vi "Init Logger.vi"(8 "error in (no error)":errorcluster, 10 "File Send Interval (Seconds)":dbl=600.0) -> (0 "error out":errorcluster, 3 "Logger out.lvclass":refnum<class "Logger.lvclass">)   [LabVIEW 2019, in "Logger.lvclass"]
uses:
  Logger.lvclass
  <vilib>/Skyline/Tag/Wrapper/Wrapper_class/Tag Value Cluster Wrapper.ctl
  <vilib>/Skyline/Configuration/Configuration_class/NI Skyline Configuration.lvclass
  <vilib>/Skyline/Tag/Shared/typedefs/Tag Value Cluster.ctl
  <vilib>/Skyline/Tag/Shared/typedefs/DataType.ctl
  <vilib>/Skyline/Tag/Wrapper/Wrapper_class/NI Skyline Tag.lvclass
  <vilib>/Skyline/Tag/Shared/typedefs/TagProperty.ctl
  Logger.lvclass/Logger.ctl
  <vilib>/Skyline/Tag/Wrapper/Wrapper AMQP_class/Open Tag AMQP.vi
  <vilib>/Skyline/Tag/Wrapper/Wrapper_class/Generate Tag Cluster (String) 2.vi
  <vilib>/Skyline/Tag/Wrapper/Wrapper_class/Generate Tag Cluster (Boolean) 2.vi
  <vilib>/Skyline/Tag/Wrapper/Wrapper_class/Generate Tag Cluster (I32) 2.vi
  <vilib>/Skyline/Message/AMQP/sync/Open (Sync).vi
  <vilib>/Skyline/Message/AMQP/NI Skyline Message AMQP (Sync).lvclass
  <vilib>/Skyline/Tag/Shared/NI Skyline Tag.lvlib
  <vilib>/Skyline/Tag/Wrapper/Wrapper AMQP_class/NI Skyline Tag AMQP.lvclass
  <vilib>/Skyline/Message/NI Skyline Message.lvclass
  <vilib>/Skyline/Utilities/NI Skyline Utilities.lvlib
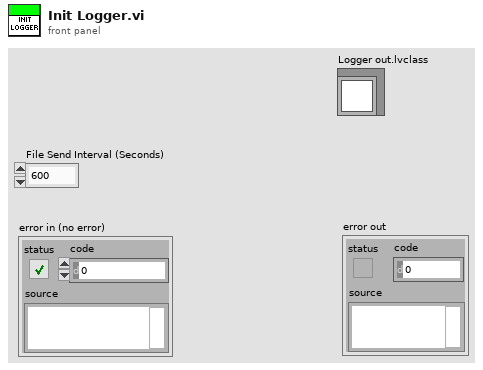
[diagram p1: front panel]
types:
  T1 = typedef "NI Skyline Tag.lvclass/Tag Value Cluster Wrapper.ctl" = cluster{"Configuration":refnum<class "NI Skyline Configuration.lvclass">, "Tag Cluster":T2}
  T2 = typedef "NI Skyline Tag.lvlib/Tag Value Cluster.ctl" = cluster{"Path":string, "Data Type":T3, "Value":string, "Time Stamp":timestamp}
  T3 = typedef "NI Skyline Tag.lvlib/DataType.ctl" = enum32{"Double", "I32", "String", "Boolean", "U64", "Timestamp"}
  T4 = typedef "NI Skyline Tag.lvlib/TagProperty.ctl" = cluster{"key":string, "value":string}
  T5 = cluster{"Tag Units":string, "Tag Path":string, "Tag Reference":refnum<class "NI Skyline Tag.lvclass">}
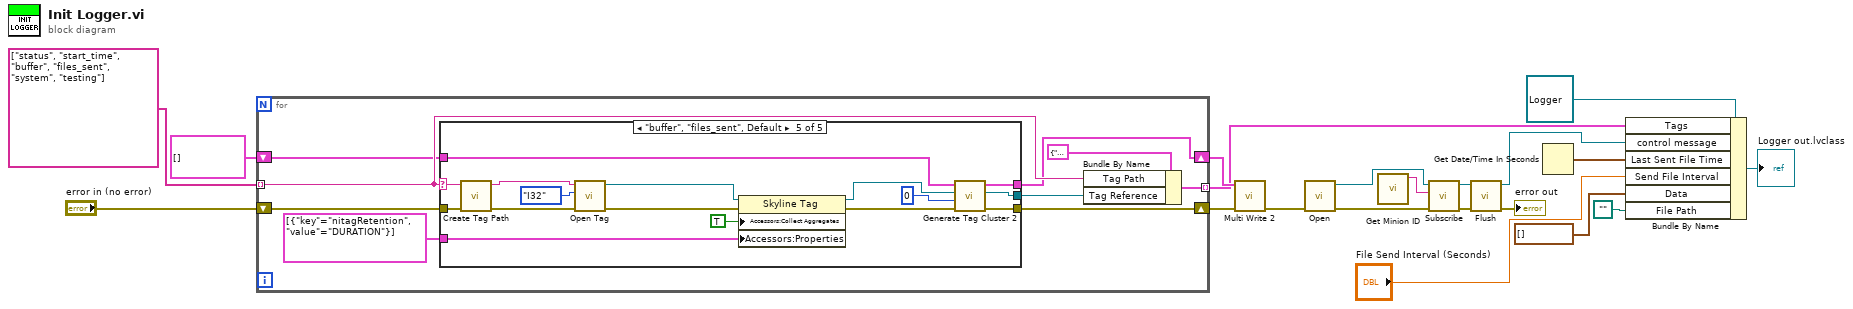
[diagram p0: block diagram]
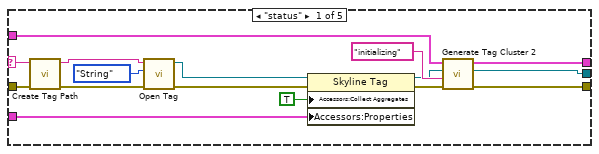
[diagram p2: hidden frame]
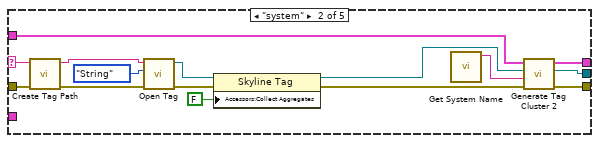
[diagram p3: hidden frame]
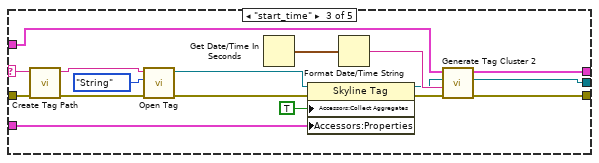
[diagram p4: hidden frame]
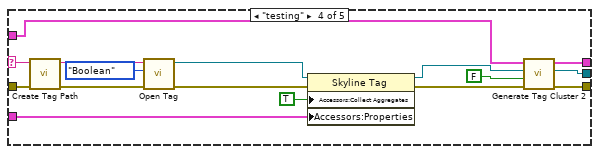
[diagram p5: hidden frame]
diagram:
  n1 = for {
    shift-right: [w29] -> w15
    shift-left: "error in (no error)" -> [w26]
    tunnel: string[] ["status", "start_time", "buffer", "files_sent", "system", "testing"] -> [w27] mode=indexing
    tunnel: [w28] -> w3 mode=indexing
    shift-right: [w22] -> w10
    shift-left: T1[] [] ("tag clusters out") -> [w23]
    n2 = case shown="\"buffer\", \"files_sent\", Default" w27 {
      selector: w27 -> [w44 w59 w62 w81 w99]
      tunnel: [w42 w57 w74 w92 w108] -> w29
      tunnel: [w43 w58 w75 w93 w109] -> w24
      tunnel: w26 -> [w45 w60 w63 w82 w98]
      tunnel: [w38 w53 w72 w90 w106] -> w22
      tunnel: w23 -> [w31 w47 w73 w91 w105]
      tunnel: T4[] [{"key"="nitagRetention", "value"="DURATION"}] ("Properties") -> [w30 _ w61 w80 w94]
      frame "status" {
        n3 = call "Create Tag Path.vi"("error in (no error)"=w45, "tag name"=w44) -> ("error out"=w41:errorcluster, "path"=w40:string)  [unwired: 8 in]
        n4 = call-poly <vilib>:"Open Tag.vi"("error in (no error)"=w41, "data type"=DataType."String" ("Data Type"), "path"=w40) -> ("error out"=w34:errorcluster, "tag"=w35:refnum<class "NI Skyline Tag.lvclass">)  [unwired: 7 in]
        n5 = property on="Property Node" class="Skyline Tag"(reference=w35, error in=w34, "Accessors:Collect Aggregates"=TRUE ("Collect Aggregates"), "Accessors:Properties"=w30) -> (reference out=w33:refnum<class "NI Skyline Tag.lvclass">, error out=w32:errorcluster)
        n6 = call-poly <vilib>:"Generate Tag Cluster 2.vi"("error in (no error)"=w32, "value"="initializing" ("string"), "tag in"=w33, "tag clusters in"=w31) -> ("error out"=w42:errorcluster, "tag out"=w43:refnum<class "NI Skyline Tag.lvclass">, "tag clusters out"=w38:T1[])  [unwired: 5 in]
      }
      frame "system" {
        n7 = call "Create Tag Path.vi"("error in (no error)"=w60, "tag name"=w59) -> ("error out"=w56:errorcluster, "path"=w55:string)  [unwired: 8 in]
        n8 = call-poly <vilib>:"Open Tag.vi"("error in (no error)"=w56, "data type"=DataType."String" ("Data Type"), "path"=w55) -> ("error out"=w50:errorcluster, "tag"=w51:refnum<class "NI Skyline Tag.lvclass">)  [unwired: 7 in]
        n9 = property on="Property Node" class="Skyline Tag"(reference=w51, error in=w50, "Accessors:Collect Aggregates"=FALSE ("Collect Aggregates")) -> (reference out=w49:refnum<class "NI Skyline Tag.lvclass">, error out=w48:errorcluster)
        n10 = call <vilib>:"Get System Name.vi"() -> ("system name"=w46:string)  [unwired: 11 in]
        n11 = call-poly <vilib>:"Generate Tag Cluster 2.vi"("error in (no error)"=w48, "value"=w46, "tag in"=w49, "tag clusters in"=w47) -> ("error out"=w57:errorcluster, "tag out"=w58:refnum<class "NI Skyline Tag.lvclass">, "tag clusters out"=w53:T1[])  [unwired: 5 in]
      }
      frame "start_time" {
        n12 = call "Create Tag Path.vi"("error in (no error)"=w63, "tag name"=w62) -> ("error out"=w64:errorcluster, "path"=w65:string)  [unwired: 8 in]
        n13 = call-poly <vilib>:"Open Tag.vi"("error in (no error)"=w64, "data type"=DataType."String" ("Data Type"), "path"=w65) -> ("error out"=w68:errorcluster, "tag"=w69:refnum<class "NI Skyline Tag.lvclass">)  [unwired: 7 in]
        n14 = Get Date/Time In Seconds() -> (seconds since 1Jan1904=w77:timestamp)
        n15 = property on="Property Node" class="Skyline Tag"(reference=w69, error in=w68, "Accessors:Collect Aggregates"=TRUE ("Collect Aggregates"), "Accessors:Properties"=w61) -> (reference out=w67:refnum<class "NI Skyline Tag.lvclass">, error out=w66:errorcluster)
        n16 = Format Date/Time String(seconds (now)=w77) -> (date/time string=w71:string)  [unwired: 2 in]
        n17 = call-poly <vilib>:"Generate Tag Cluster 2.vi"("error in (no error)"=w66, "value"=w71, "tag in"=w67, "tag clusters in"=w73) -> ("error out"=w74:errorcluster, "tag out"=w75:refnum<class "NI Skyline Tag.lvclass">, "tag clusters out"=w72:T1[])  [unwired: 5 in]
      }
      frame "testing" {
        n18 = call "Create Tag Path.vi"("error in (no error)"=w82, "tag name"=w81) -> ("error out"=w83:errorcluster, "path"=w84:string)  [unwired: 8 in]
        n19 = call-poly <vilib>:"Open Tag.vi"("error in (no error)"=w83, "data type"=DataType."Boolean", "path"=w84) -> ("error out"=w87:errorcluster, "tag"=w88:refnum<class "NI Skyline Tag.lvclass">)  [unwired: 7 in]
        n20 = property on="Property Node" class="Skyline Tag"(reference=w88, error in=w87, "Accessors:Collect Aggregates"=TRUE ("Collect Aggregates"), "Accessors:Properties"=w80) -> (reference out=w86:refnum<class "NI Skyline Tag.lvclass">, error out=w85:errorcluster)
        n21 = call-poly <vilib>:"Generate Tag Cluster 2.vi"("error in (no error)"=w85, "value"=FALSE, "tag in"=w86, "tag clusters in"=w91) -> ("error out"=w92:errorcluster, "tag out"=w93:refnum<class "NI Skyline Tag.lvclass">, "tag clusters out"=w90:T1[])  [unwired: 5 in]
      }
      frame "buffer", "files_sent", Default {
        n22 = call "Create Tag Path.vi"("error in (no error)"=w98, "tag name"=w99) -> ("error out"=w97:errorcluster, "path"=w96:string)  [unwired: 8 in]
        n23 = call-poly <vilib>:"Open Tag.vi"("error in (no error)"=w97, "data type"=DataType."I32", "path"=w96) -> ("error out"=w103:errorcluster, "tag"=w104:refnum<class "NI Skyline Tag.lvclass">)  [unwired: 7 in]
        n24 = property on="Property Node" class="Skyline Tag"(reference=w104, error in=w103, "Accessors:Collect Aggregates"=TRUE ("Collect Aggregates"), "Accessors:Properties"=w94) -> (reference out=w101:refnum<class "NI Skyline Tag.lvclass">, error out=w100:errorcluster)
        n25 = call-poly <vilib>:"Generate Tag Cluster 2.vi"("error in (no error)"=w100, "value"=0, "tag in"=w101, "tag clusters in"=w105) -> ("error out"=w108:errorcluster, "tag out"=w109:refnum<class "NI Skyline Tag.lvclass">, "tag clusters out"=w106:T1[])  [unwired: 5 in]
      }
    }
    n26 = Bundle By Name(cluster=T5 {"Tag Units"="", "Tag Path"="", "Tag Reference"=refnum} ("Tag"), "Tag Path"=w27, "Tag Reference"=w24) -> (w28:T5)
  }
  n27 = call <vilib>:"Multi Write 2.vi"("error in (no error)"=w15, "tag clusters"=w10) -> ("error out"=w14:errorcluster)  [unwired: 9 in]
  n28 = call-poly <vilib>:"Open.vi"("error in (no error)"=w14) -> ("error out"=w8:errorcluster, "message session"=w9:refnum<class "NI Skyline Message AMQP (Sync).lvclass">)  [unwired: 9 in]
  n29 = call <vilib>:"Get Minion ID.vi"() -> ("minion id"=w4:string)  [unwired: 11 in]
  n30 = call-dynamic "Subscribe.vi"("error in (no error)"=w8, "topic"=w4, "message session in"=w9) -> ("error out"=w7:errorcluster, "message session out"=w6:refnum<class "NI Skyline Message AMQP (Sync).lvclass">)  [unwired: 7 in]
  n31 = call-dynamic "Flush.vi"("error in (no error)"=w7, "sync message session in"=w6) -> ("error out"=→"error out":errorcluster, "sync message session out"=w13:refnum<class "NI Skyline Message AMQP (Sync).lvclass">)  [unwired: 8 in]
  n32 = Get Date/Time In Seconds() -> (seconds since 1Jan1904=w18:timestamp)
  n33 = Bundle By Name(cluster=refnum<class "Logger.lvclass"> refnum ("Logger out.lvclass"), "Tags"=w3, "control message"=w13, "Last Sent File Time"=w18, "Send File Interval"="File Send Interval (Seconds)", "Data"=waveform(dbl)[] [], "File Path"=path "") -> (→"Logger out.lvclass":refnum<class "Logger.lvclass">)
